vi "Exit Refs.vi"(8 "error in (no error)":errorcluster, 11 "Queue in (NaN)":refnum<queue>) -> (0 "error out":errorcluster, 1 "Registered Queues":refnum<queue>[](array[refnum]), 2 "Exit SEQ":refnum<queue>, 3 "Exit User Event":refnum<user-event>)   [LabVIEW 2018, in "Exit.lvlib"]
uses:
  Exit.lvlib
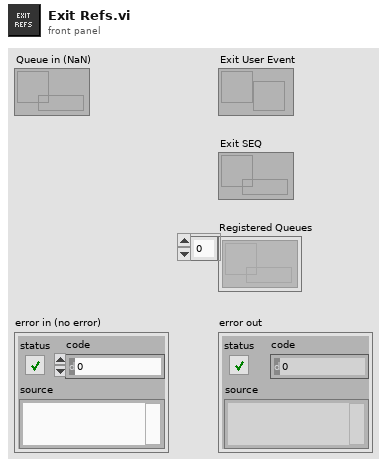
[diagram p1: front panel]
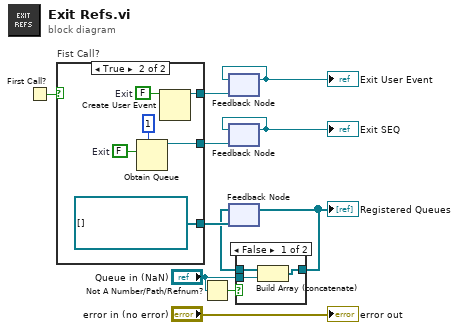
[diagram p0: block diagram]
diagram:
  n1 = First Call?() -> (First Call?: T/F=w9:bool)
  n2 = case "Fist Call?" shown="True" w9 {
    tunnel: [_ w12] -> w11
    tunnel: [_ w16] -> w8
    tunnel: [_ refnum<queue>[] [] ("Queue in")] -> w7
    frame False {
    }
    frame True {
      w14 = FALSE  # Exit
      w17 = FALSE  # Exit
      n3 = Obtain Queue(max queue size (-1, unlimited)=1, element data type=w14) -> (queue out=w12:refnum<queue>)  [unwired: 3 in, 2 out]
      n4 = Create User Event(user event datatype=w17) -> (user event=w16:refnum<user-event>)  [unwired: 1 in, 1 out]
    }
  }
  n5 = Not A Number/Path/Refnum?(number/path/refnum="Queue in (NaN)") -> (NaN/Path/Refnum?=w2:bool)
  n6 = feedback #1(w8) -> (w1:refnum<user-event>)
  "Exit User Event" <- w1
  n7 = feedback-in #1(w1) -> ()
  n8 = feedback #2(w11) -> (w10:refnum<queue>)
  "Exit SEQ" <- w10
  n9 = feedback-in #2(w10) -> ()
  n10 = feedback #3(w7) -> (w5:refnum<queue>[])
  n11 = case shown="False" w2 {
    tunnel: "Queue in (NaN)" -> [w20 _]
    tunnel: w5 -> [w19 w21]
    tunnel: [w18 w21] -> w4
    frame False {
      n12 = Build Array (concatenate)(w19, w20) -> (w18:refnum<queue>[])
    }
    frame True {
    }
  }
  "Registered Queues" <- w4
  n13 = feedback-in #3(w4) -> ()
  "error out" <- "error in (no error)"
